vi "GetTerminal.vi"(6 "error in":errorcluster, 9 "Local in":refnum<class "Local.lvclass">) -> (0 "error out":errorcluster, 3 "Local out":refnum<class "Local.lvclass">, 4 "terminal":refnum<class "Terminal.lvclass">)   [LabVIEW 2014, in "Raspberry Pi Compatible Compiler for LabVIEW.lvlib" / "Local.lvclass"]
uses:
  Local.lvclass
  Terminal/Terminal.lvclass
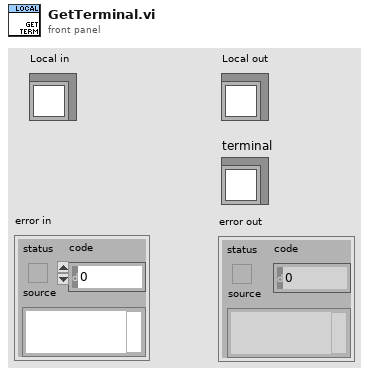
[diagram p1: front panel]
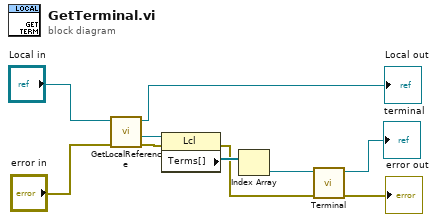
[diagram p0: block diagram]
diagram:
  n1 = call "GetLocalReference.vi"("error in"="error in", "Local in"="Local in") -> ("error out"=w6:errorcluster, "reference out"=w7:refnum<vi>, "Local out"=→"Local out":refnum<class "Local.lvclass">)  [unwired: 7 in]
  n2 = property class="Lcl"(reference=w7, error in=w6) -> (error out=w4:errorcluster, "Terms[]"=w5:refnum<vi>[])  [unwired: 1 out]
  n3 = Index Array(array=w5) -> (element=w3:refnum<vi>)  [unwired: 1 in]
  n4 = call "Terminal.vi"("error in"=w4, "refnum"=w3) -> ("error out"=→"error out":errorcluster, "terminal"=→"terminal":refnum<class "Terminal.lvclass">)  [unwired: 8 in]
